vi "ReadPAQtags.vi"(8 "error in (no error)":errorcluster, 11 "DBAL in":refnum<class "DBAL.lvclass">) -> (0 "error out":errorcluster, 2 "PAQ_TAGs":T1 {"TAGprop"."TagFunc" format="%08x"; "TAGprop"."RangeL" format="%.2f"; "TAGprop"."RangeH" format="%.2f"}, 3 "DBAL out":refnum<class "DBAL.lvclass">)   [LabVIEW 2020, in "Sgraph_lib_V1.lvlib" / "DBAL.lvclass"]
doc: "Read the PAQ Qtype TAG properties from the database"
uses:
  DBAL.lvclass
  controls/DBAL_TAGprops.ctl
  controls/DBAL_TAGpropEdit.ctl
  Common/controls/typedef_com_TagProp.ctl
  Builds/Sgraph_lib_V1.lvlib
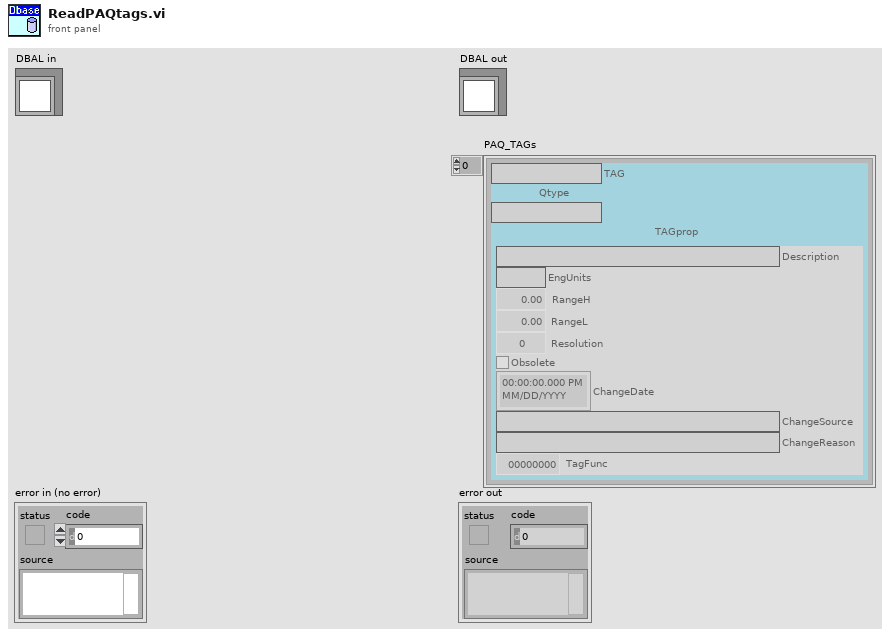
[diagram p1: front panel]
types:
  T1 = typedef "Sgraph_lib_V1.lvlib/DBAL_TAGprops.ctl" = T2[]
  T2 = typedef "Sgraph_lib_V1.lvlib/DBAL_TAGpropEdit.ctl" = cluster{"TAG":string, "Qtype":string, "TAGprop":T3}
  T3 = typedef "Sgraph_lib_V1.lvlib/typedef_com_TagProp.ctl" = cluster{"Description":string, "EngUnits":string, "RangeH":dbl, "RangeL":dbl, "Resolution":i32, "Obsolete":bool, "ChangeDate":timestamp, "ChangeSource":string, "ChangeReason":string, "TagFunc":u32}
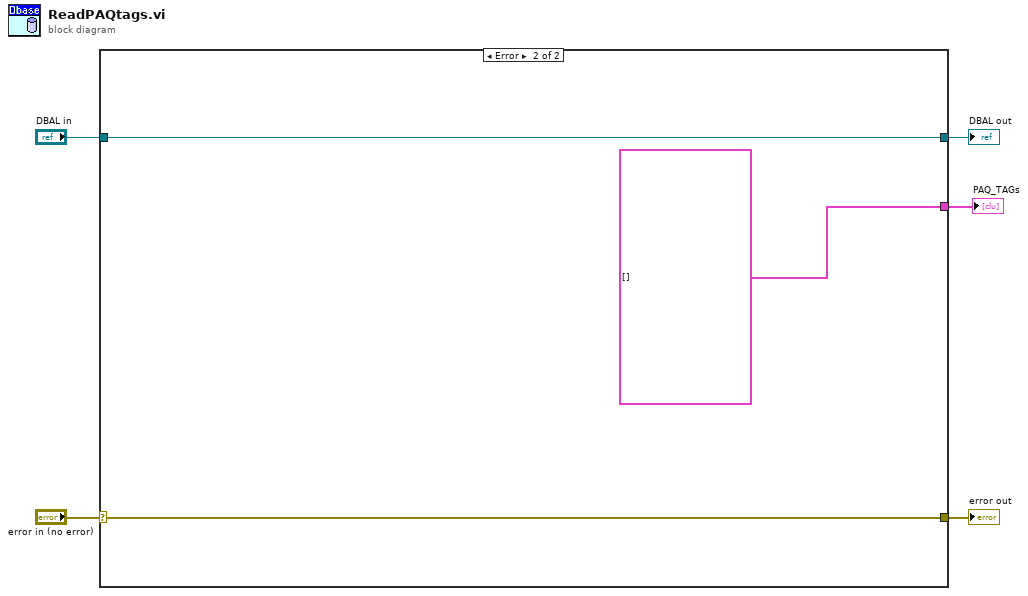
[diagram p0: block diagram]
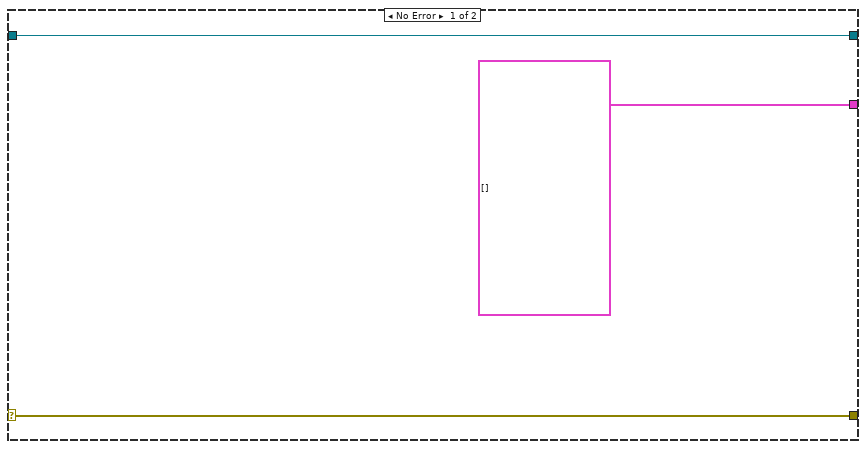
[diagram p2: hidden frame]
diagram:
  n1 = case shown="Error" "error in (no error)" {
    selector: "error in (no error)" -> [w7 w11]
    tunnel: [w7 w11] -> w4
    tunnel: [w8 w10] -> w2
    tunnel: "DBAL in" -> [w8 w10]
    tunnel: [T2[] [] ("PAQ_TAGs") T1 [] ("PAQ_TAGs")] -> w1
    frame No Error {
    }
    frame Error {
    }
  }
  "error out" <- w4
  "DBAL out" <- w2
  "PAQ_TAGs" <- w1
